vi "ENVIO_DATOS_AURAWHEEL.vi"(6 "timestamp":dbl, 7 "Array TAGs 2":string[](array[string]), 8 "error AURA":errorcluster, 9 "Max RMS Ruedas":dbl[][](array[numeric]), 10 "p_sp 2":dbl, 11 "p_tp 2":dbl) -> (0 "error out":errorcluster)   [LabVIEW 2015]
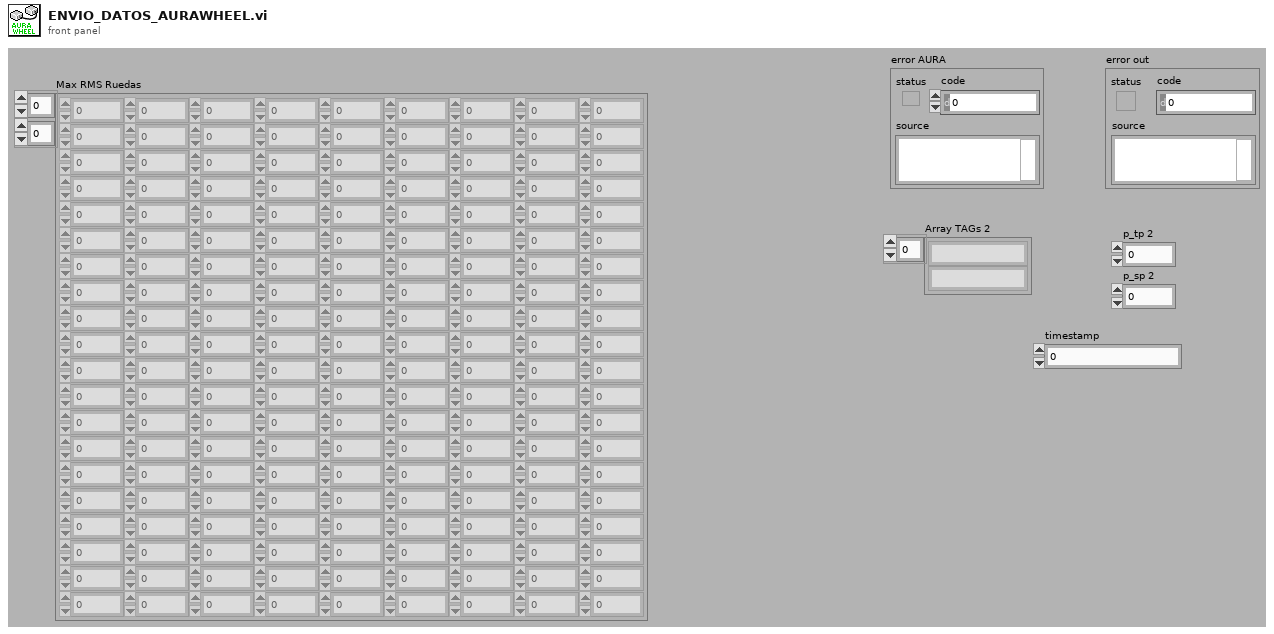
[diagram p1: front panel]
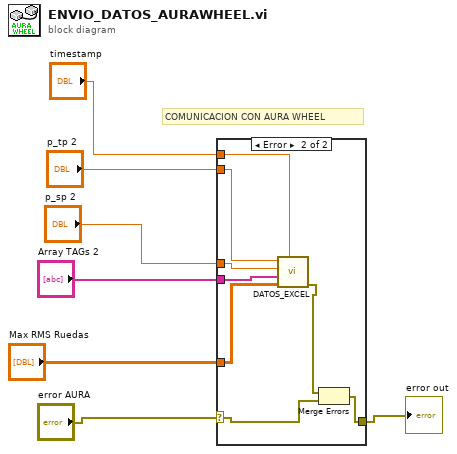
[diagram p0: block diagram]
diagram:
  # "COMUNICACION CON AURA WHEEL"
  n1 = case shown="Error" "error AURA" {
    selector: "error AURA" -> [w8 w10]
    tunnel: [w8 w9] -> w6
    tunnel: "p_sp 2" -> [_ w16]
    tunnel: "p_tp 2" -> [_ w15]
    tunnel: "Array TAGs 2" -> [_ w14]
    tunnel: "Max RMS Ruedas" -> [_ w13]
    tunnel: "timestamp" -> [_ w12]
    frame No Error {
    }
    frame Error {
      n2 = call "DATOS_EXCEL.vi"("timestamp"=w12, "Max RMS Ruedas"=w13, "Array TAGs 2"=w14, "p_sp 2"=w16, "p_tp 2"=w15) -> ("error out"=w11:errorcluster)  [unwired: 6 in]
      n3 = Merge Errors(w11, w10) -> (w9:errorcluster)
    }
  }
  "error out" <- w6
